vi "Receive DBL Value Msg.vi"(8 "error in (no error)":errorcluster, 10 "DBLValueMsg":refnum<class "DBLValueMsg.lvclass">, 11 "TopLevelApplication in":refnum<class "TopLevelApplication.lvclass">) -> (0 "error out":errorcluster, 3 "TopLevelApplication out":refnum<class "TopLevelApplication.lvclass">)   [LabVIEW 2015, in "TopLevelApplication.lvlib" / "TopLevelApplication.lvclass"]
uses:
  TopLevelApplication.lvclass
  AutoRegistration/ActorAutoRegistration Messages/DBLValueMsg/DBLValueMsg.lvclass
  Dialog Box Implementations/OneButtonDialogBox/OneButtonDialogBox.lvclass
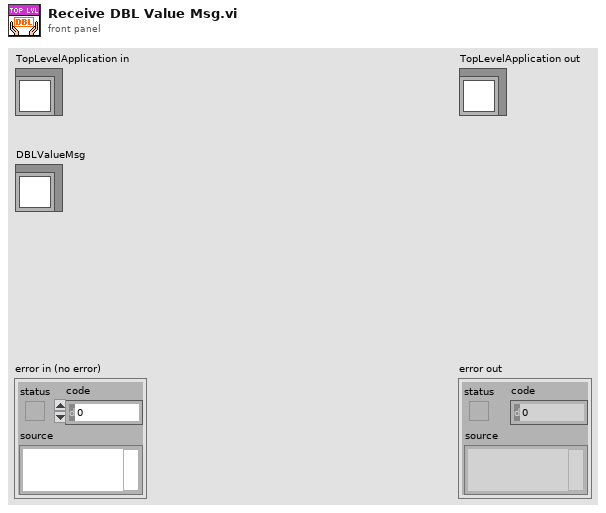
[diagram p1: front panel]
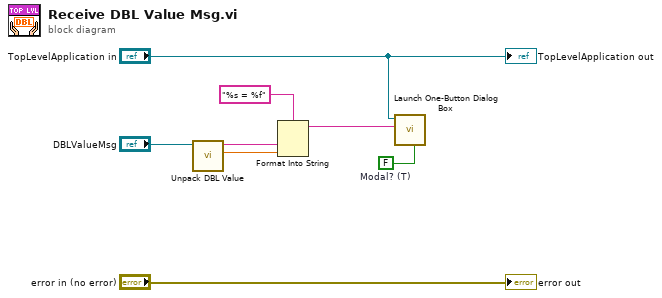
[diagram p0: block diagram]
diagram:
  w1 = FALSE  # Modal? (T)
  n1 = call-dynamic "Unpack DBL Value.vi"("DBLValueMsg in"="DBLValueMsg") -> ("Value"=w5:dbl, "Name"=w6:string)  [unwired: 9 in]
  n2 = Format Into String(format string="%s = %f", w6, w5) -> (resulting string=w2:string)  [unwired: 2 in, 1 out]
  n3 = call "Launch One-Button Dialog Box.vi"("Modal? (T)"=w1, "Message Text"=w2, "Dialog Launcher"="TopLevelApplication in") -> ()  [unwired: 8 in, 1 out]
  "error out" <- "error in (no error)"
  "TopLevelApplication out" <- "TopLevelApplication in"
